vi "GUI_Slink.vi"() -> ()   [LabVIEW 2013]
uses:
  Device Drivers/Gentec Slink/sclae_typdef.ctl
  Shared/Device Driver/OnOffTypeDef.ctl
  Shared/GUI_Template/GUI_master/tcp_new_data_event.ctl
  Shared/GUI_Template/GUI_master/tcp new data cluster.ctl
panel:
  out "tcp data event 2":T1
  in  "Tab Control":enum32{"Control", "History"}(tab)=enum."History"
  in  "Reading.Channel 1::1":dbl=0.001 caption="Ch1 (J)" min=0.0 max=0.0 format="%_3p"
  in  "Reading.Channel 2::1":dbl=0.001 caption="Ch2 (J)" min=0.0 max=0.0 format="%_3p"
  in  "Scale.Channel 1::1":T2 caption="Scale Ch1"
  in  "Scale.Channel 2::1":T2 caption="Scale Ch2"
  in  "trigger.Channel 1::1":T3 caption="Trigger Channel 1"
  in  "trigger.Channel 2::1":T3 caption="trigger Channel 2"
  in  "Refresh Button":bool
  out "Device name":string
  in  "stop":bool
  out "Ch1 2":cluster{dbl[], dbl[]}[](graph)
  out "Ch1":cluster{dbl[], dbl[]}[](graph)
  in  "Clear":bool
  in  "Select device":string(combo)="LB_EnergyMeter_1"
  out "GUIdevice 1":string="LB_EnergyMeter_1"
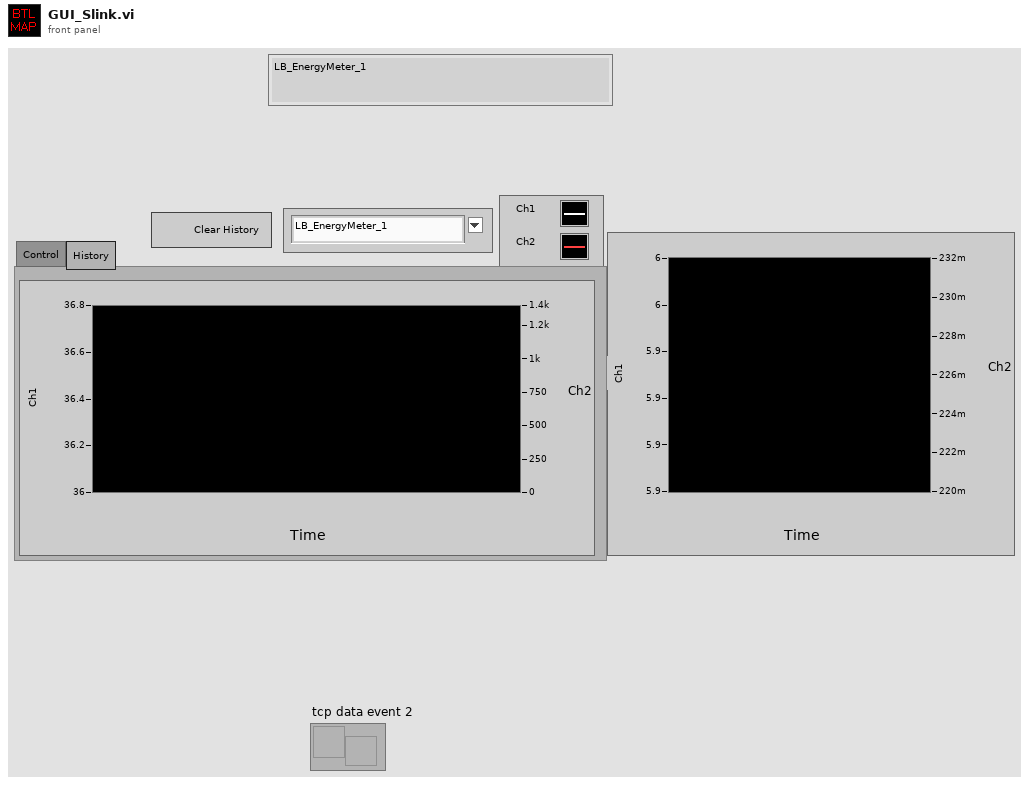
[diagram p1: front panel]
types:
  T1 = typedef "tcp_new_data_event.ctl" = refnum<user-event>
  T2 = typedef "sclae_typdef.ctl" = enum16{"1p", "3p", "10p", "30p", "100p", "300p", "1n", "3n", "10n", "30n", "100n", "300n", "1u", "3u", "10u", "30u", "100u", "300u", "1m", "3m", "10m", "30m", "100m", "300m", "1", "3", "10", "30", "100", "300", "1k", "3k", "10k", "30k", "100k", "300k", "1meg", "3meg", "10meg", "30meg", "100meg", "300meg"}
  T3 = typedef "OnOffTypeDef.ctl" = enum16{"off", "on"}
  T4 = enum32{"invalid app kind", "Development System", "Run Time System", "Student Edition", "Embedded LabVIEW", "Evaluation", "Custom"}
  T5 = typedef "tcp new data cluster.ctl" = cluster{"EventEnum":enum16{"new data", "connection status update"}, "Device name":string}
  T6 = enum32{"Invalid", "Standard", "Closed", "Hidden", "Minimized", "Maximized"}
  T7 = cluster{"Core":cluster{"Current VI Reference":refnum<vi>, "Close Panel on Exit?":bool}, "Your Boolean data":bool, "Your string data":string, "SuperGUI":cluster{"STOP queue":refnum<queue>, "SuperGUI ref":refnum<vi>, "event reg":refnum<event-registration>}, "Timer":u32}
  T8 = cluster{"STOP queue":refnum<queue>, "SuperGUI ref":refnum<vi>, "event reg":refnum<event-registration>}
  T9 = cluster{"Current VI Reference":refnum<vi>, "Close Panel on Exit?":bool}
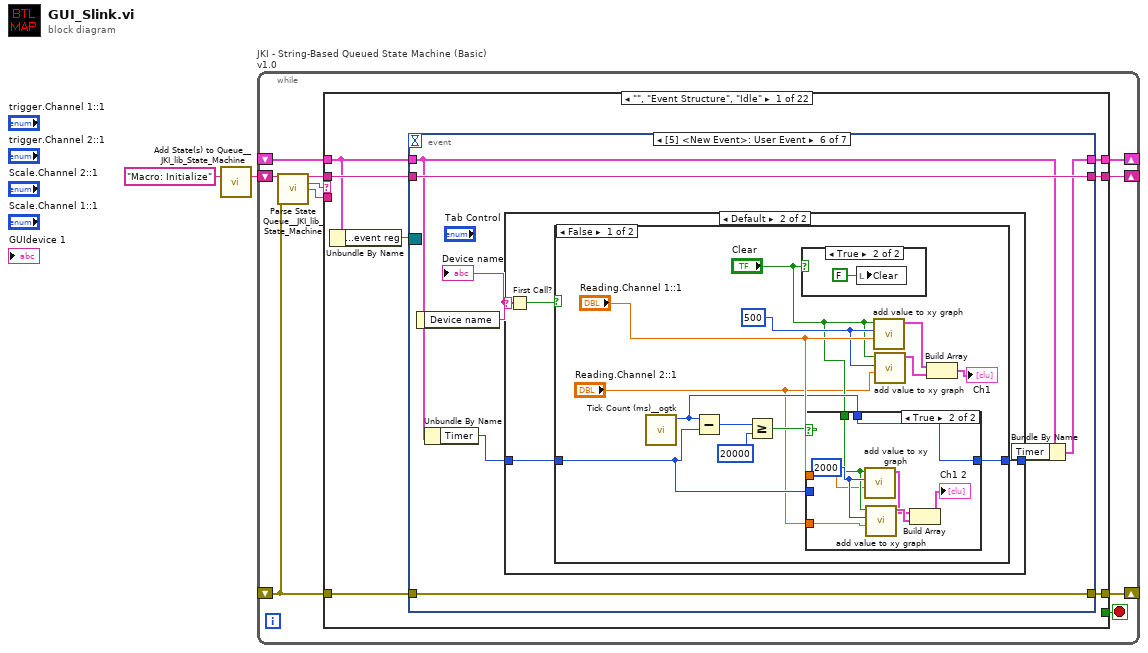
[diagram p0: block diagram]
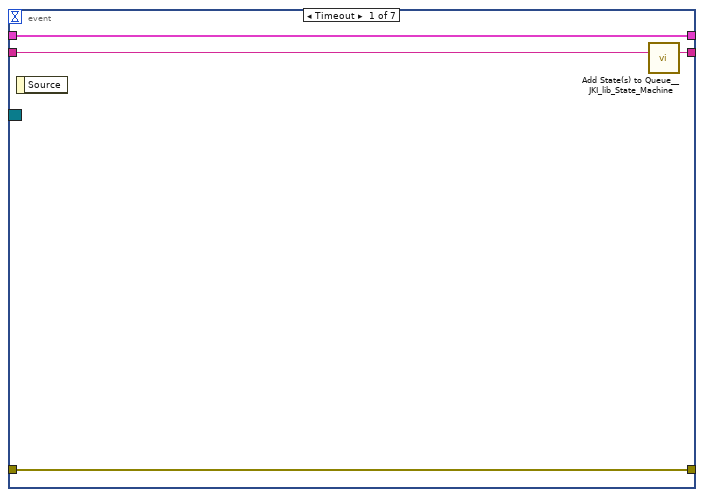
[diagram p2: hidden frame]
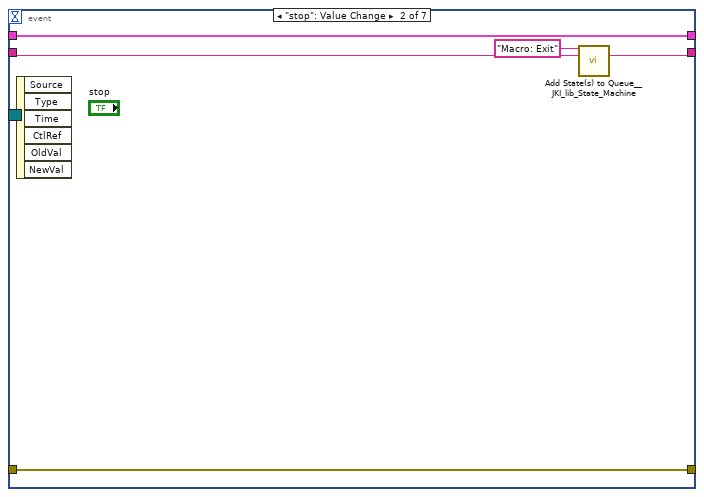
[diagram p3: hidden frame]
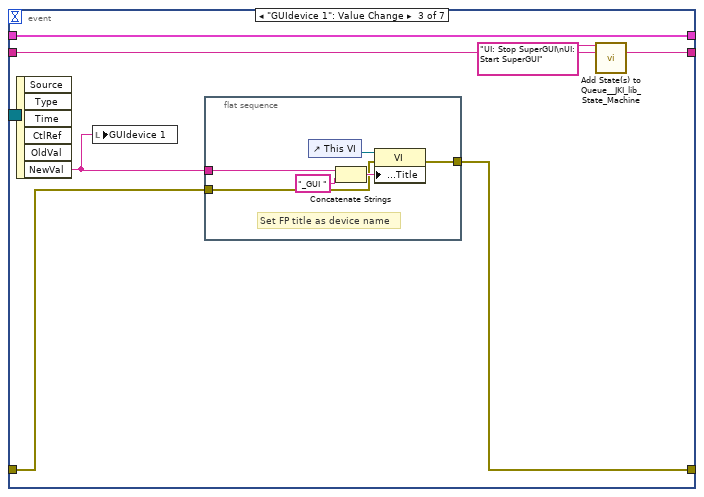
[diagram p4: hidden frame]
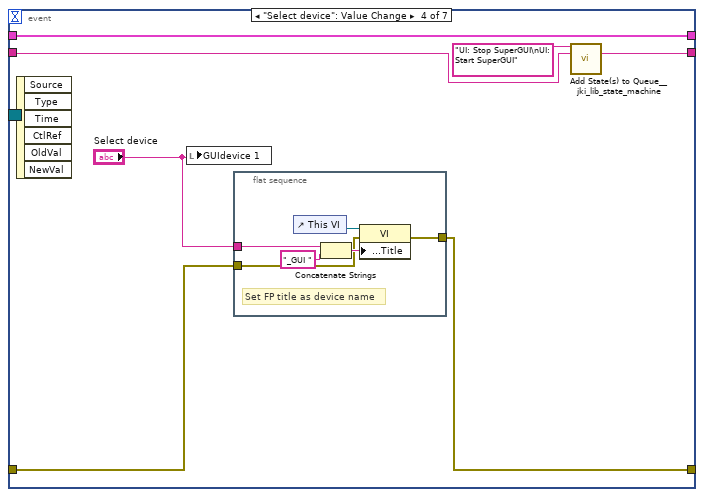
[diagram p5: hidden frame]
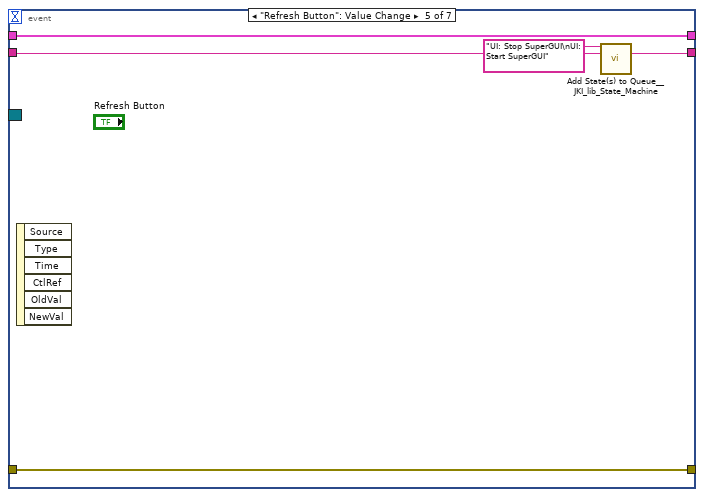
[diagram p6: hidden frame]
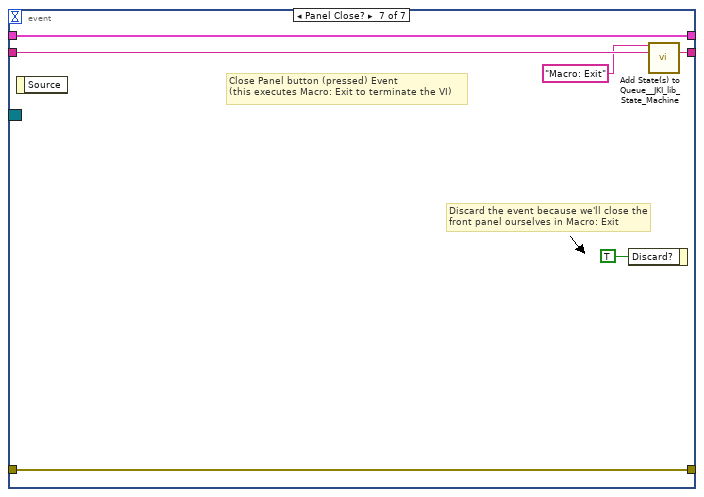
[diagram p11: hidden frame]
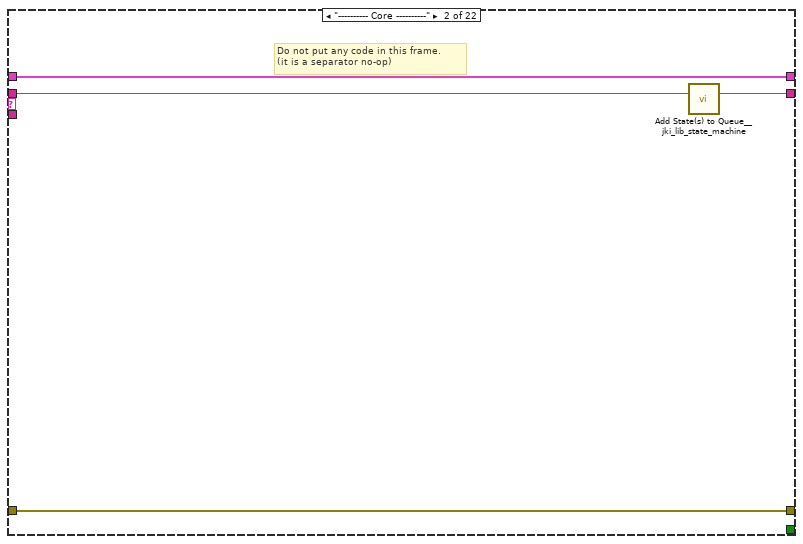
[diagram p12: hidden frame]
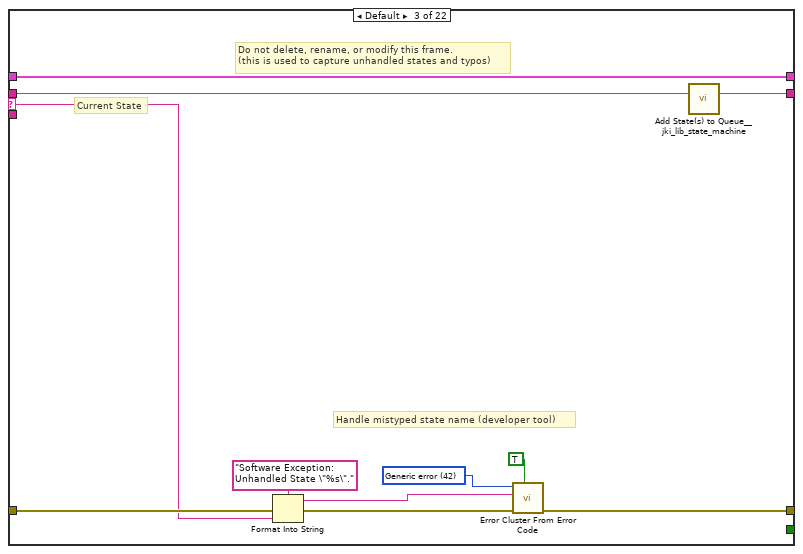
[diagram p13: hidden frame]
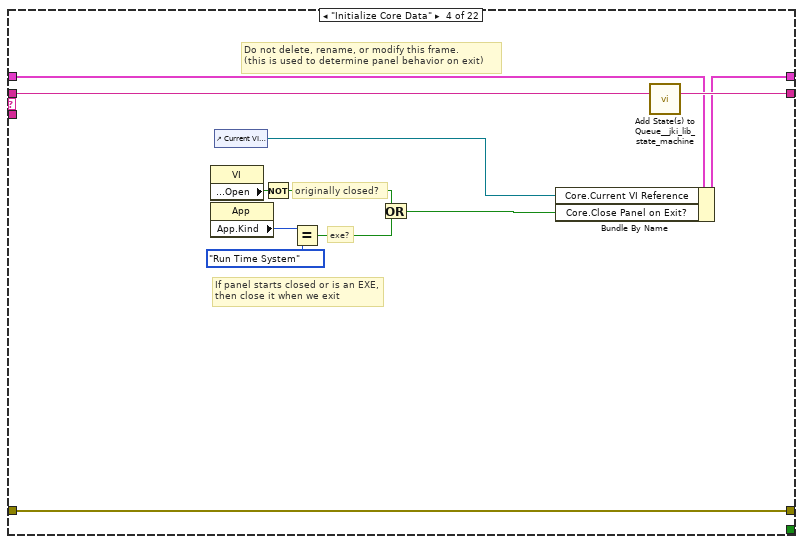
[diagram p14: hidden frame]
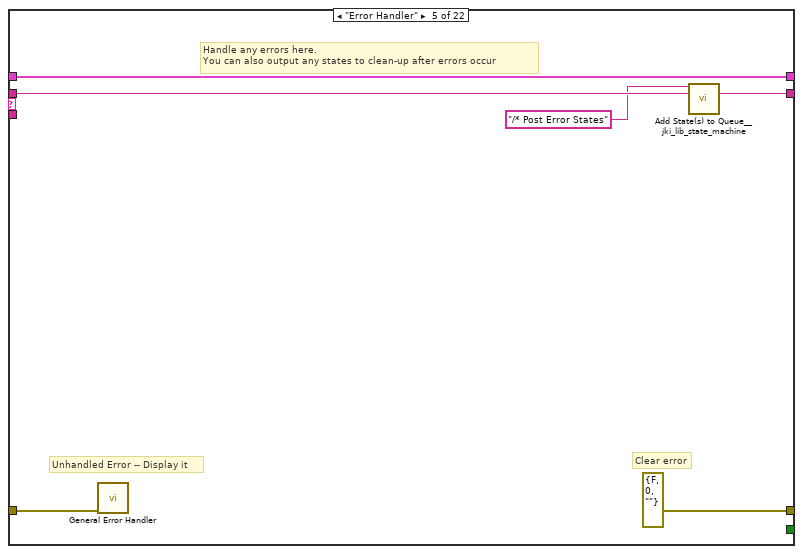
[diagram p15: hidden frame]
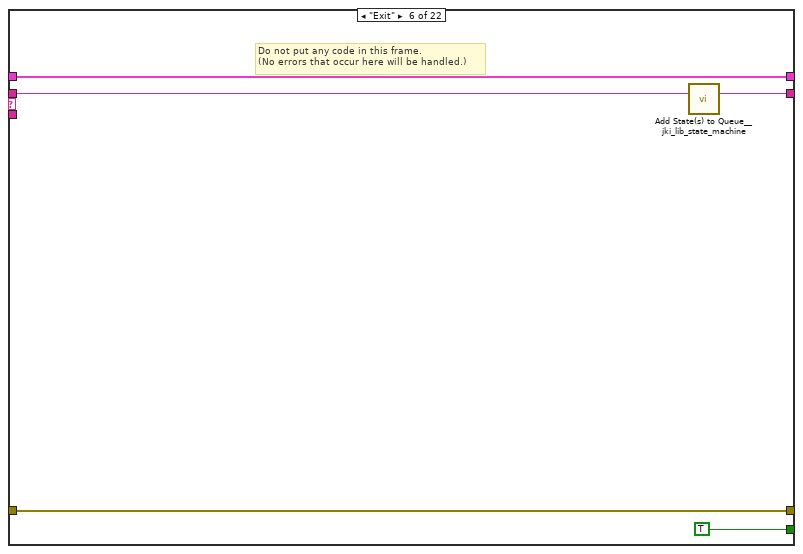
[diagram p16: hidden frame]
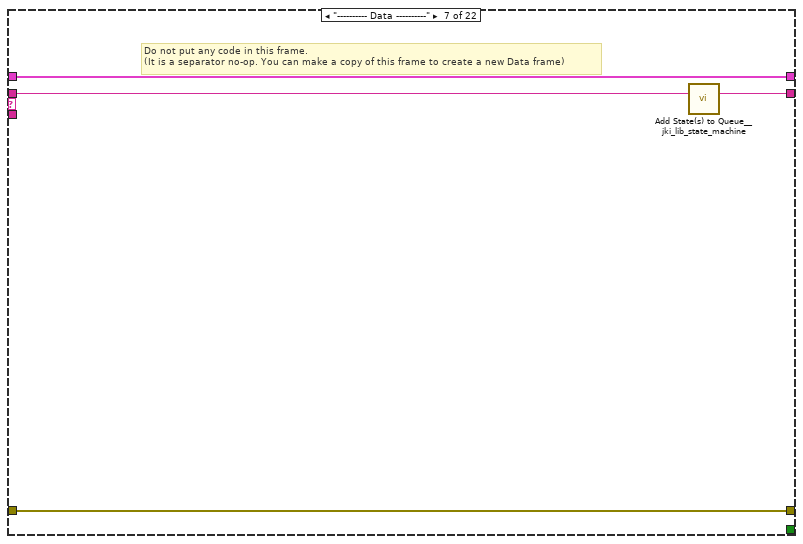
[diagram p17: hidden frame]
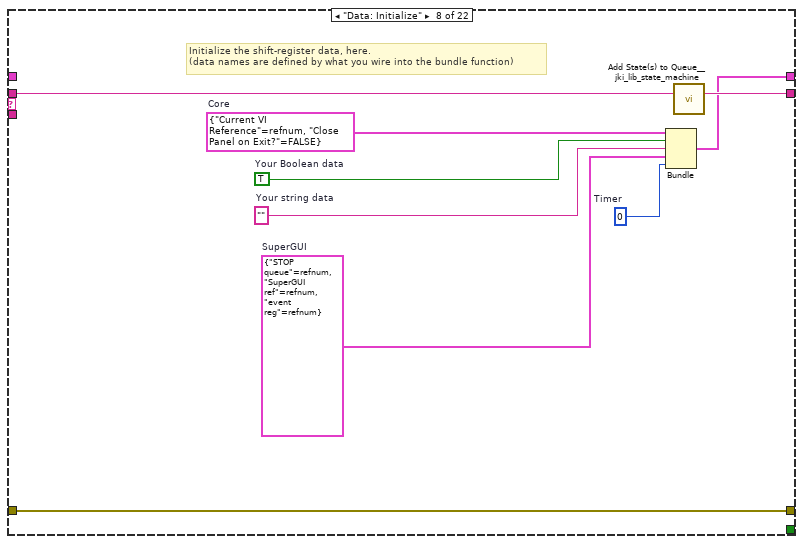
[diagram p18: hidden frame]
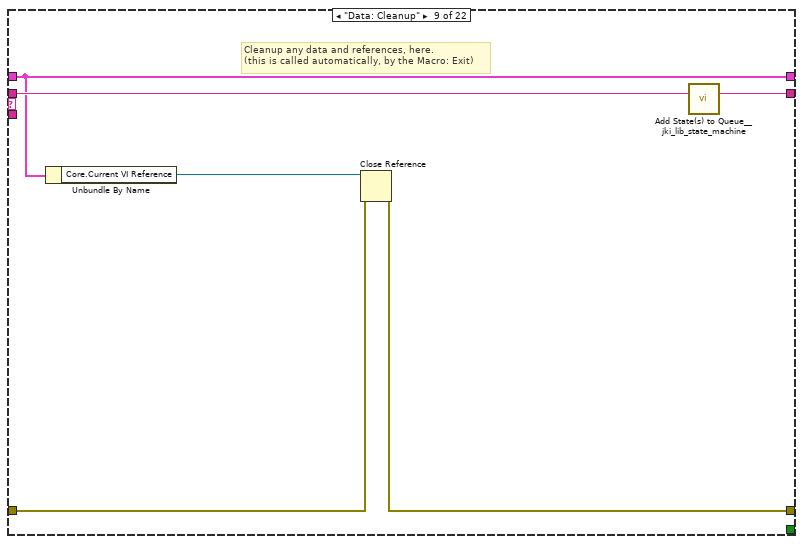
[diagram p19: hidden frame]
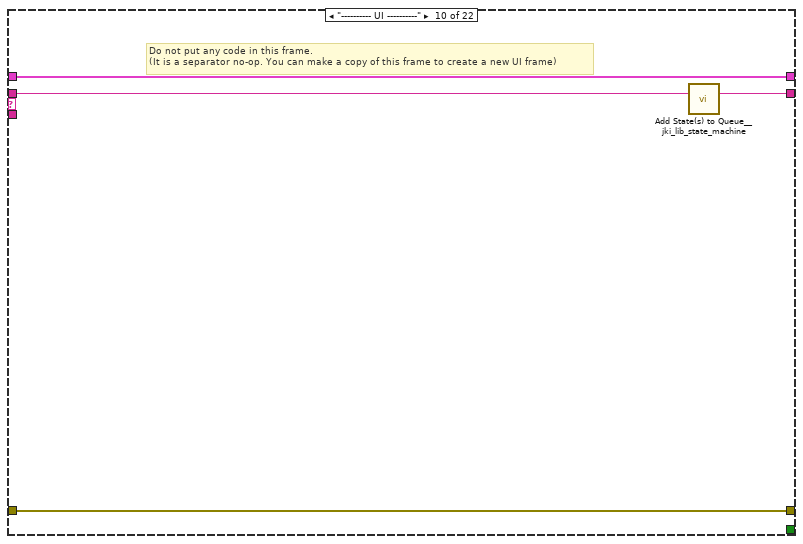
[diagram p20: hidden frame]
diagram:
  n1 = call <vilib>:"Add State(s) to Queue__JKI_lib_State_Machine.vi"("State(s) in (\"\")"="Macro: Initialize") -> ("States Out"=w2:string)  [unwired: 14 in]
  n2 = while "JKI - String-Based Queued State Machine (Basic) v1.0" {
    shift-right: [w5] -> _
    shift-left: _ -> [w4]
    shift-right: [w8] -> _
    shift-left: _ -> [w3]
    shift-right: [w7] -> _
    shift-left: w2 -> [w9]
    stop <- w6 stop-if-true
    n3 = call <vilib>:"Parse State Queue__JKI_lib_State_Machine.vi"("State Queue"=w9, "Error In (no error)"=w3) -> ("Remaining States"=w11:string, "Current State"=w12:string, "Arguments"=w10:string)  [unwired: 11 in]
    n4 = case shown="\"\", \"Event Structure\", \"Idle\"" w12 {
      selector: w12 -> [_ _ w105 _ _ _ _ _ _ _ _ _ _ _ _ _ _ _ _ _ _ _]
      tunnel: w11 -> [w19 w104 w109 w127 w133 w138 w142 w151 w157 w161 w171 w177 w213 w221 w227 w238 w264 w269 w279 w283 w287 w291]
      tunnel: w10 -> [_ _ _ _ _ _ _ _ _ _ _ _ _ _ w222 w232 _ _ _ _ _ _]
      tunnel: w4 -> [w14 w101 w107 w118 w130 w136 w139 _ w152 w158 w164 w175 w204 w216 w225 w234 w261 w266 w276 w280 w284 w288]
      tunnel: [w17 w102 w111 w124 errorcluster {"status"=FALSE, "code"=0, "source"=""} ("error out") w135 w140 w148 w153 w159 w168 w172 w197 w214 w223 w235 w262 w267 w277 w281 w285 w289] -> w8
      tunnel: w3 -> [w16 w102 w110 w124 w129 w135 w140 w148 w154 w159 w169 w173 w198 w215 w224 w236 w262 w267 w277 w281 w285 w289]
      tunnel: [w18 w103 w108 w126 w132 w137 w141 w150 w156 w160 w170 w176 w212 w220 w226 w237 w263 w268 w278 w282 w286 w290] -> w7
      tunnel: [_ _ _ _ _ TRUE _ _ _ _ _ _ _ _ _ _ _ _ _ _ _ _] -> w6
      tunnel: [w15 w101 w107 w125 w130 w136 w139 w149 w152 w158 w163 w175 w203 w216 w225 w234 w261 w266 w276 w280 w284 w288] -> w5
      frame "", "Event Structure", "Idle" {
        n5 = Unbundle By Name(w14) -> ("SuperGUI.event reg"=w13:refnum<event-registration>)
        n6 = event shown="[5] <New Event>: User Event" {
          selector: w13 -> [_ _ _ _ _ _ _]
          dyn-events: _ -> [_ _ _ _ _ _ _]
          timeout: _ -> [_ _ _ _ _ _ _]
          tunnel: w19 -> [w23 w26 w32 w44 w57 w66 w100]
          tunnel: [w22 w25 w31 w43 w56 w66 w99] -> w18
          tunnel: w14 -> [w20 w28 w35 w48 w59 w61 w97]
          tunnel: [w21 w27 w33 w46 w58 w65 w98] -> w17
          tunnel: w16 -> [w21 w27 w34 w47 w58 w65 w98]
          tunnel: [w20 w28 w35 w48 w59 w60 w97] -> w15
          event Timeout {
            n7 = event-data() -> ()  [unwired: 1 in, 1 out]
            n8 = call <vilib>:"Add State(s) to Queue__JKI_lib_State_Machine.vi"("State(s) in (\"\")"=w23) -> ("States Out"=w22:string)  [unwired: 14 in]
          }
          event "stop": Value Change {
            n9 = event-data() -> ()  [unwired: 1 in, 6 out]
            n10 = call <vilib>:"Add State(s) to Queue__JKI_lib_State_Machine.vi"("State(s) in Front (\"\")"="Macro: Exit", "State(s) in (\"\")"=w26) -> ("States Out"=w25:string)  [unwired: 13 in]
          }
          event "GUIdevice 1": Value Change {
            n11 = event-data() -> ("NewVal"=w29:string)  [unwired: 1 in, 5 out]
            n12 = local write "GUIdevice 1"(w29) -> ()
            n13 = flat-sequence {
              tunnel: [w38] -> w33
              tunnel: w34 -> [w37]
              tunnel: w29 -> [w36]
              frame #0 {
                # "Set FP title as device name"
                n14 = control-ref of="This VI"() -> (w41:refnum<vi>)
                n15 = Concatenate Strings(w36, "_GUI ") -> (w40:string)
                n16 = property class="VI"(reference=w41, error in=w37, "Front Panel.Title"=w40) -> (error out=w38:errorcluster)  [unwired: 1 out]
              }
            }
            n17 = call <vilib>:"Add State(s) to Queue__JKI_lib_State_Machine.vi"("State(s) in Front (\"\")"="UI: Stop SuperGUI\nUI: Start SuperGUI", "State(s) in (\"\")"=w32) -> ("States Out"=w31:string)  [unwired: 13 in]
          }
          event "Select device": Value Change {
            n18 = event-data() -> ()  [unwired: 1 in, 6 out]
            n19 = local write "GUIdevice 1"("Select device") -> ()
            n20 = flat-sequence {
              tunnel: [w51] -> w46
              tunnel: w47 -> [w50]
              tunnel: "Select device" -> [w49]
              frame #0 {
                # "Set FP title as device name"
                n21 = control-ref of="This VI"() -> (w54:refnum<vi>)
                n22 = Concatenate Strings(w49, "_GUI ") -> (w53:string)
                n23 = property class="VI"(reference=w54, error in=w50, "Front Panel.Title"=w53) -> (error out=w51:errorcluster)  [unwired: 1 out]
              }
            }
            n24 = call <vilib>:"Add State(s) to Queue__jki_lib_state_machine.vi"("State(s) in Front (\"\")"="UI: Stop SuperGUI\nUI: Start SuperGUI", "State(s) in (\"\")"=w44) -> ("States Out"=w43:string)  [unwired: 13 in]
          }
          event "Refresh Button": Value Change {
            n25 = event-data() -> ()  [unwired: 1 in, 6 out]
            n26 = call <vilib>:"Add State(s) to Queue__JKI_lib_State_Machine.vi"("State(s) in Front (\"\")"="UI: Stop SuperGUI\nUI: Start SuperGUI", "State(s) in (\"\")"=w57) -> ("States Out"=w56:string)  [unwired: 13 in]
          }
          event User Event {
            n27 = event-data() -> ("Device name"=w64:string)  [unwired: 1 in]
            "Device name" <- w64
            n28 = Unbundle By Name(w61) -> ("Timer"=w63:u32)
            n29 = case shown="Default" w64 {
              tunnel: w63 -> [w67 w69]
              tunnel: [w67 w68] -> w62
              frame "" {
              }
              frame Default {
                n30 = First Call?() -> (First Call?: T/F=w70:bool)
                n31 = case shown="False" w70 {
                  tunnel: w69 -> [w77 w94]
                  tunnel: [w79 w94] -> w68
                  frame False {
                    w76 = 500 ("max points")
                    n32 = call <userlib>:"Tick Count (ms)__ogtk.vi"() -> ("millisecond timer value"=w78:u32)  [unwired: 10 in, 1 out]
                    n33 = Subtract(x=w78, y=w77) -> (x-y=w82:u32)
                    n34 = Greater Or Equal?(x=w82, y=u32 20000 ("min time between updates")) -> (x >= y?=w80:bool)
                    n35 = case shown="True" "Clear" {
                      frame False {
                      }
                      frame True {
                        n36 = local write "Clear"(FALSE ("Clear")) -> ()
                      }
                    }
                    n37 = case shown="True" w80 {
                      tunnel: "Reading.Channel 1::1" -> [_ w86]
                      tunnel: [w84 w92] -> w79
                      tunnel: w78 -> [_ w92]
                      tunnel: w77 -> [w84 _]
                      tunnel: "Clear" -> [_ w90]
                      tunnel: "Reading.Channel 2::1" -> [_ w85]
                      frame False {
                      }
                      frame True {
                        w91 = 2000 ("max points")
                        n38 = call "add value to xy graph.vi"("new value"=w86, "max points"=w91, "Wire in Stop To Clear Graph on Each Run"=w90) -> ("XY Graph"=w88:cluster{dbl[], dbl[]})  [unwired: 8 in]
                        n39 = call "add value to xy graph.vi"("new value"=w85, "max points"=w91, "Wire in Stop To Clear Graph on Each Run"=w90) -> ("XY Graph"=w89:cluster{dbl[], dbl[]})  [unwired: 8 in]
                        n40 = Build Array(w88, w89) -> (→"Ch1 2":cluster{dbl[], dbl[]}[])
                      }
                    }
                    n41 = call "add value to xy graph.vi"("new value"="Reading.Channel 1::1", "max points"=w76, "Wire in Stop To Clear Graph on Each Run"="Clear") -> ("XY Graph"=w74:cluster{dbl[], dbl[]})  [unwired: 8 in]
                    n42 = call "add value to xy graph.vi"("new value"="Reading.Channel 2::1", "max points"=w76, "Wire in Stop To Clear Graph on Each Run"="Clear") -> ("XY Graph"=w73:cluster{dbl[], dbl[]})  [unwired: 8 in]
                    n43 = Build Array(w74, w73) -> (→"Ch1":cluster{dbl[], dbl[]}[])
                  }
                  frame True {
                  }
                }
              }
            }
            n44 = Bundle By Name(cluster=w61, "Timer"=w62) -> (w60:T7)
          }
          event Panel Close? {
            # "Discard the event because we'll close the front panel ourselves in Macro: Exit"
            # "Close Panel button (pressed) Event\n(this executes Macro: Exit to terminate the VI)"
            n45 = event-data() -> ()  [unwired: 1 in, 1 out]
            n46 = event-data("Discard?"=TRUE) -> ()  [unwired: 1 in, 1 out]
            n47 = call <vilib>:"Add State(s) to Queue__JKI_lib_State_Machine.vi"("State(s) in Front (\"\")"="Macro: Exit", "State(s) in (\"\")"=w100) -> ("States Out"=w99:string)  [unwired: 13 in]
          }
        }
      }
      frame "---------- Core ----------" {
        # "Do not put any code in this frame.\n(it is a separator no-op)"
        n48 = call <vilib>:"Add State(s) to Queue__jki_lib_state_machine.vi"("State(s) in (\"\")"=w104) -> ("States Out"=w103:string)  [unwired: 14 in]
      }
      frame Default {
        w114 = 42 items=["No error", "Argument error", "Memory is full", "Out of zone", "End of file", "File already open", "Generic file I/O error", "File not found", "File permission error", "Disk is full", "Duplicate path", "Too many files open", "System feature not enabled", "Resource file not found", "Cannot add resource", "Resource not found", "Image not found", "Image memory error", "Pen does not exist", "Config type invalid", "Config token not found", "Config parse error", "Config memory error", "Bad external code format", "Bad external code offset", "External code not present", "Null window", "Destroy window error", "Null menu", "Print aborted", "Bad print record", "Print driver error", "Windows error during printing", "Memory error during printing", "Print dialog error", "Generic print error", "Invalid device refnum", "Device not found", "Device parameter error", "Device unit error", "Cannot open device", "Device call aborted", "Generic error", "Cancelled by user", "Object ID too low", "Object ID too high", "Object not in heap", "Unknown heap", "Unknown object (invalid DefProc)", "Unknown object (DefProc not in table)", "Message out of range", "Invalid (null) method", "Unknown message", "Manager call not supported", "Bad address", "Network operation in progress", "Network operation timed out", "Connection is busy", "Network attribute not supported", "Network error", "Address in use", "System out of memory", "Connection aborted", "Connection refused", "Not connected", "Already connected", "Connection closed", "Initialization error (interapplication manager)", "Bad occurrence", "Wait on unbound occurrence handler", "Occurrence queue overflow", "Datalog type conflict", "Unused", "Unrecognized type (interapplication manager)", "Memory corrupt", "Failed to make temporary DLL", "Old CIN version", "Drag socket not found", "Failed to load drop-object", "Failed to register OLE object", "Failed to release OLE object", "Format specifier type mismatch", "Unknown format specifier", "Too few format specifiers", "Too many format specifiers", "Scan failed", "Newer CIN version", "Error converting to variant", "Runtime menu error", "Password tampered", "Variant attribute not found", "Incompatible variant data type", "Event data is not available", "Event Store is not present", "Occurrence is not found", "Event Queue is not created", "Event info is not available", "Refnum passed is NULL", "Error retrieving Class GUID", "Error retrieving CoClass GUID", "Error retrieving TypeLib GUID.", "Bad built application magic bytes.", "Specific driver is different from the specific driver associated with the Logical Name.", "There is no session opened to the class driver.", "Max Error", "MAX - Error with config objects", "MAX - Error loading configuration", "MAX - Group not supported"]
        # "Current State"
        # "Do not delete, rename, or modify this frame.\n(this is used to capture unhandled states and typos)"
        # "Handle mistyped state name (developer tool)"
        n49 = Format Into String(format string="Software Exception: Unhandled State \"%s\"." ("message"), error in=w110, w105) -> (resulting string=w113:string, error out=w112:errorcluster)  [unwired: 1 in]
        n50 = call <vilib>:"Error Cluster From Error Code.vi"("show call chain? (False)"=TRUE, "error in (no error)"=w112, "error message (\"\")"=w113, "error code (0)"=w114) -> ("error out"=w111:errorcluster)  [unwired: 5 in]
        n51 = call <vilib>:"Add State(s) to Queue__jki_lib_state_machine.vi"("State(s) in (\"\")"=w109) -> ("States Out"=w108:string)  [unwired: 14 in]
      }
      frame "Initialize Core Data" {
        # "Do not delete, rename, or modify this frame.\n(this is used to determine panel behavior on exit)"
        # "originally closed?"
        # "exe?"
        # "If panel starts closed or is an EXE, then close it when we exit"
        n52 = property class="VI"() -> ("Front Panel.Open"=w123:bool)  [unwired: 2 in, 2 out]
        n53 = property class="App"() -> ("App.Kind"=w122:T4)  [unwired: 2 in, 2 out]
        n54 = control-ref of="Current VI Reference"() -> (w116:refnum<vi>)
        n55 = Not(x=w123) -> (.not. x?=w120:bool)
        n56 = Equal?(x=w122, y=T4."Run Time System" ("Application:Kind")) -> (x = y?=w119:bool)
        n57 = Or(x=w120, y=w119) -> (x .or. y?=w117:bool)
        n58 = Bundle By Name(cluster=w118, "Core.Current VI Reference"=w116, "Core.Close Panel on Exit?"=w117) -> (w125:T7)
        n59 = call <vilib>:"Add State(s) to Queue__jki_lib_state_machine.vi"("State(s) in (\"\")"=w127) -> ("States Out"=w126:string)  [unwired: 14 in]
      }
      frame "Error Handler" {
        # "Unhandled Error -- Display it"
        # "Handle any errors here.\nYou can also output any states to clean-up after errors occur"
        # "Clear error"
        n60 = call <vilib>:"General Error Handler.vi"("error in (no error)"=w129) -> ()  [unwired: 10 in, 5 out]
        n61 = call <vilib>:"Add State(s) to Queue__jki_lib_state_machine.vi"("State(s) in Front (\"\")"="/* Post Error States", "State(s) in (\"\")"=w133) -> ("States Out"=w132:string)  [unwired: 13 in]
      }
      frame "Exit" {
        # "Do not put any code in this frame.\n(No errors that occur here will be handled.)"
        n62 = call <vilib>:"Add State(s) to Queue__jki_lib_state_machine.vi"("State(s) in (\"\")"=w138) -> ("States Out"=w137:string)  [unwired: 14 in]
      }
      frame "---------- Data ----------" {
        # "Do not put any code in this frame.\n(It is a separator no-op. You can make a copy of this frame to create a new Data frame)"
        n63 = call <vilib>:"Add State(s) to Queue__jki_lib_state_machine.vi"("State(s) in (\"\")"=w142) -> ("States Out"=w141:string)  [unwired: 14 in]
      }
      frame "Data: Initialize" {
        w143 = u32 0  # Timer
        w144 = T8 {"STOP queue"=refnum, "SuperGUI ref"=refnum, "event reg"=refnum}  # SuperGUI
        w145 = T9 {"Current VI Reference"=refnum, "Close Panel on Exit?"=FALSE}  # Core
        w147 = TRUE  # Your Boolean data
        w146 = ""  # Your string data
        # "Initialize the shift-register data, here.\n(data names are defined by what you wire into the bundle function)"
        n64 = Bundle("Core"=w145, "Your Boolean data"=w147, "Your string data"=w146, "SuperGUI"=w144, "Timer"=w143) -> (w149:T7)  [unwired: 1 in]
        n65 = call <vilib>:"Add State(s) to Queue__jki_lib_state_machine.vi"("State(s) in (\"\")"=w151) -> ("States Out"=w150:string)  [unwired: 14 in]
      }
      frame "Data: Cleanup" {
        # "Cleanup any data and references, here.\n(this is called automatically, by the Macro: Exit)"
        n66 = Unbundle By Name(w152) -> ("Core.Current VI Reference"=w155:refnum<vi>)
        n67 = Close Reference(reference=w155, error in (no error)=w154) -> (error out=w153:errorcluster)
        n68 = call <vilib>:"Add State(s) to Queue__jki_lib_state_machine.vi"("State(s) in (\"\")"=w157) -> ("States Out"=w156:string)  [unwired: 14 in]
      }
      frame "---------- UI ----------" {
        # "Do not put any code in this frame.\n(It is a separator no-op. You can make a copy of this frame to create a new UI frame)"
        n69 = call <vilib>:"Add State(s) to Queue__jki_lib_state_machine.vi"("State(s) in (\"\")"=w161) -> ("States Out"=w160:string)  [unwired: 14 in]
      }
      frame "UI: Initialize" {
        # "Initialize the User Interface, here.\n(this is called automatically, by the Macro: Init)"
        n70 = call <userlib>:"Fit VI window to Largest Dec__ogtk.vi"("error in (no error)"=w169) -> ("error out"=w168:errorcluster)  [unwired: 5 in, 1 out]
        n71 = local read "GUIdevice 1"() -> (w165:string)
        n72 = call "getDevices.vi"("Device Class"="Gentec Slink") -> ("All Devices"=w166:string[])
        n73 = property on="Select device" class="CmbBox"("Strings[]"=w166, "Value"=w165) -> ()  [unwired: 2 in, 2 out]
        n74 = call <userlib>:"Tick Count (ms)__ogtk.vi"() -> ("millisecond timer value"=w162:u32)  [unwired: 10 in, 1 out]
        n75 = Bundle By Name(cluster=w164, "Timer"=w162) -> (w163:T7)
        n76 = call <vilib>:"Add State(s) to Queue__jki_lib_state_machine.vi"("State(s) in (\"\")"=w171) -> ("States Out"=w170:string)  [unwired: 14 in]
      }
      frame "UI: Get Device Name" {
        # "Initialize the User Interface, here.\n(this is called automatically, by the Macro: Init)"
        n77 = First Call?() -> (First Call?: T/F=w174:bool)
        n78 = case shown="True" w174 {
          tunnel: w173 -> [w178 w180]
          tunnel: [w178 w179] -> w172
          frame False {
          }
          frame True {
            n79 = disable-structure "Get Device name from control for vi mode\nand command line arg for exe" shown="RUN_TIME_ENGINE==True" {
              disable-tunnel: w180 -> [w181 w183]
              disable-tunnel: [w181 w182] -> w179
              frame condition #0 (active) {
              }
              frame condition #1 {
                n80 = control-ref of="This Application"() -> (w191:refnum<vi>)
                n81 = property class="App"(reference=w191) -> ("App.Args"=w190:string[])  [unwired: 1 in, 2 out]
                n82 = Index Array(array=w190, index #1=1 ("index")) -> (element #1=w184:string)  [unwired: 2 in, 2 out]
                n83 = Empty String/Path?(string/path=w184) -> (empty?=w188:bool)
                n84 = control-ref of="This VI"() -> (w187:refnum<vi>)
                n85 = case shown="False" w188 {
                  tunnel: w184 -> [w192 _]
                  frame False {
                    n86 = local write "GUIdevice 1"(w192) -> ()
                  }
                  frame True {
                  }
                }
                n87 = Concatenate Strings(w184, "_GUI ") -> (w186:string)
                n88 = property class="VI"(reference=w187, error in=w183, "Front Panel.Title"=w186) -> (error out=w182:errorcluster)  [unwired: 1 out]
              }
            }
          }
        }
        n89 = call <vilib>:"Add State(s) to Queue__jki_lib_state_machine.vi"("State(s) in (\"\")"=w177) -> ("States Out"=w176:string)  [unwired: 14 in]
      }
      frame "UI: Start SuperGUI" {
        # "create stop queue for supergui and its clones"
        # "x100 abort will be dependent on caller VI\nx80 abort will be independent of caller vi, this will abort vi when labview is closed."
        # "Start SuperGUI asynchronous way"
        n90 = vi-ref "GUI_Master_subvi_reentrant_queues.vi"() -> (w196:refnum<vi>)
        n91 = property class="VI"(reference=w196) -> ("Path"=w195:path)  [unwired: 1 in, 2 out]
        n92 = Create User Event(user event datatype=T5 {"EventEnum"=enum."new data", "Device name"="Device name"} ("New Event"), error in=w198) -> (user event=w199:refnum<user-event>, error out=w205:errorcluster)
        "tcp data event 2" <- w199
        n93 = control-ref of="This Application"() -> (w202:refnum<vi>)
        n94 = control-ref of="This VI"() -> (w201:refnum<vi>)
        n95 = Open VI Reference(type specifier VI Refnum (for type only)=refnum<vi> refnum, vi path=w195, options=256) -> (vi reference=w211:refnum<vi>, error out=w210:errorcluster)  [unwired: 3 in]
        n96 = register-events(w199) -> (reference out=w193:refnum<event-registration>)  [unwired: 2 in, 1 out]
        n97 = call "supergui create stop queue.vi"() -> ("STOP Queue out"=w207:refnum<queue>)  [unwired: 11 in]
        n98 = Current VI's Menubar() -> (w200:refnum<k9>)
        n99 = call-by-ref "Start Asynchronous Call"(reference=w211, error in=w210, "STOP Queue in"=w207, "This Application"=w202, 8:"error in (no error)"=w205, "tcp data event"=w199, "Caller menu reference"=w200, "Caller VI ref"=w201) -> (reference out=w194:refnum<vi>, error out=w197:errorcluster)  [unwired: 5 in, 1 out]
        n100 = Bundle By Name(cluster=w204, "SuperGUI.event reg"=w193, "SuperGUI.SuperGUI ref"=w194, "SuperGUI.STOP queue"=w207) -> (w203:T7)
        n101 = call <vilib>:"Add State(s) to Queue__jki_lib_state_machine.vi"("State(s) in (\"\")"=w213) -> ("States Out"=w212:string)  [unwired: 14 in]
      }
      frame "UI: Stop SuperGUI" {
        # "Stop Supergui Clone and wait until it exit properly"
        n102 = Unbundle By Name(w216) -> ("SuperGUI.SuperGUI ref"=w218:refnum<vi>, "SuperGUI.STOP queue"=w217:refnum<queue>)
        n103 = Release Queue(queue=w217, error in (no error)=w215) -> (error out=w219:errorcluster)  [unwired: 1 in, 2 out]
        n104 = call-by-ref "Wait On Asynchronous Call"(reference=w218, error in=w219) -> ("error out"=w214:errorcluster)  [unwired: 11 in, 2 out]
        n105 = call <vilib>:"Add State(s) to Queue__jki_lib_state_machine.vi"("State(s) in (\"\")"=w221) -> ("States Out"=w220:string)  [unwired: 14 in]
      }
      frame "UI: Cursor Set" {
        # "Argument"
        # "Set and Unset Cursor Busy.\n(Usage: \"UI: Cursor Set >> Busy|Idle\")"
        n106 = case shown="\"Idle\", Default" w222 {
          tunnel: w224 -> [w229 w231]
          tunnel: [w228 w230] -> w223
          frame "Idle", Default {
            n107 = call <vilib>:"Unset Busy.vi"("error in (no error)"=w229) -> ("error out"=w228:errorcluster)  [unwired: 10 in]
          }
          frame "Busy" {
            n108 = call <vilib>:"Set Busy.vi"("error in (no error)"=w231) -> ("error out"=w230:errorcluster)  [unwired: 9 in, 1 out]
          }
        }
        n109 = call <vilib>:"Add State(s) to Queue__jki_lib_state_machine.vi"("State(s) in (\"\")"=w227) -> ("States Out"=w226:string)  [unwired: 14 in]
      }
      frame "UI: Front Panel State" {
        # "Argument"
        # "Set Front Panel Open or Closed\n(Usage: \"UI: Front Panel State >> Open|Close\")"
        n110 = Unbundle By Name(w234) -> ("Core.Current VI Reference"=w233:refnum<vi>)
        n111 = case shown="\"Open\", Default" w232 {
          tunnel: w236 -> [w242 w255]
          tunnel: [w244 w256] -> w235
          tunnel: w233 -> [w243 w253]
          frame "Open", Default {
            n112 = property class="VI"(reference=w243, error in=w242) -> (reference out=w240:refnum<vi>, error out=w241:errorcluster, "Front Panel.Open"=w239:bool)
            n113 = case shown="False" w239 {
              tunnel: [w247 w250] -> w244
              tunnel: w241 -> [w246 w250]
              tunnel: w240 -> [w245 _]
              frame False {
                n114 = invoke class="VI" method="FP.Open"(reference=w245, error in=w246, "Activate"=TRUE, "State"=T6."Standard") -> (error out=w247:errorcluster)  [unwired: 1 in, 4 out]
              }
              frame True {
              }
            }
          }
          frame "Close" {
            n115 = property class="VI"(reference=w253, error in=w255) -> (reference out=w252:refnum<vi>, error out=w254:errorcluster, "Front Panel.Open"=w251:bool)
            n116 = case shown="True" w251 {
              tunnel: [w257 w260] -> w256
              tunnel: w254 -> [w257 w259]
              tunnel: w252 -> [_ w258]
              frame False {
              }
              frame True {
                n117 = invoke class="VI" method="FP.Close"(reference=w258, error in=w259) -> (error out=w260:errorcluster)  [unwired: 1 in, 2 out]
              }
            }
          }
        }
        n118 = call <vilib>:"Add State(s) to Queue__jki_lib_state_machine.vi"("State(s) in (\"\")"=w238) -> ("States Out"=w237:string)  [unwired: 14 in]
      }
      frame "---------- Macro ----------" {
        # "Do not put any code in this frame.\n(It is a separator no-op. You can make a copy of this frame to create a new Macro frame)"
        n119 = call <vilib>:"Add State(s) to Queue__jki_lib_state_machine.vi"("State(s) in (\"\")"=w264) -> ("States Out"=w263:string)  [unwired: 14 in]
      }
      frame "Macro: Initialize" {
        # "Initialization Macro\n(This is called once, when the VI starts)"
        n120 = call <vilib>:"Add State(s) to Queue__jki_lib_state_machine.vi"("State(s) in Front (\"\")"="Data: Initialize\nInitialize Core Data\nUI: Initialize\nUI: Get Device Name\nUI: Start SuperGUI\nUI: Front Panel State >> Open", "State(s) in (\"\")"=w269) -> ("States Out"=w268:string)  [unwired: 13 in]
      }
      frame "Macro: Exit" {
        # "Exit Macro\n(This is called once, when the VI exits)"
        n121 = Unbundle By Name(w276) -> ("Core.Close Panel on Exit?"=w275:bool)
        n122 = Select(t="UI: Front Panel State >> Close", s=w275, f="") -> (s? t:f=w272:string)
        n123 = call <vilib>:"Add State(s) to Queue__jki_lib_state_machine.vi"("State(s) in (\"\")"=w272, "State(s) at Back (\"\")"="Data: Cleanup\nExit") -> ("States Out"=w270:string)  [unwired: 13 in]
        n124 = call <vilib>:"Add State(s) to Queue__jki_lib_state_machine.vi"("State(s) in Front (\"\")"=w270, "State(s) in (\"\")"=w279) -> ("States Out"=w278:string)  [unwired: 13 in]
      }
      frame "---------- New Category ----------" {
        # "Template Separator\n(You can make a copy of, or modify, this frame)"
        n125 = call <vilib>:"Add State(s) to Queue__jki_lib_state_machine.vi"("State(s) in (\"\")"=w283) -> ("States Out"=w282:string)  [unwired: 14 in]
      }
      frame "New Category: 1" {
        # "Your code here.\n(You can make a copy of, or modify, this frame)"
        n126 = call <vilib>:"Add State(s) to Queue__jki_lib_state_machine.vi"("State(s) in (\"\")"=w287) -> ("States Out"=w286:string)  [unwired: 14 in]
      }
      frame "New Category: 2" {
        # "Your code here.\n(You can make a copy of, or modify, this frame)"
        n127 = call <vilib>:"Add State(s) to Queue__jki_lib_state_machine.vi"("State(s) in (\"\")"=w291) -> ("States Out"=w290:string)  [unwired: 14 in]
      }
    }
  }
